vi "welcome.vi"() -> ()   [LabVIEW 2017]
uses:
  GLOBAL/auto.vi
  GLOBAL/all vi close.vi
panel:
  out "first time direct auto":bool
  in  "error in":errorcluster
  in  "EXIT":bool
  in  "PRINTER":bool
  in  "REPORT":bool
  in  "MAIN":bool
  in  "DATA":bool
  in  "USER":bool
  in  "COUNTER":bool
  in  "SETTING":bool
  in  "SHIFT SETTING":bool
  in  "LOGIN":bool
  # "TRACEABILITY"
  # "Powered By- NI Vision, Pune"
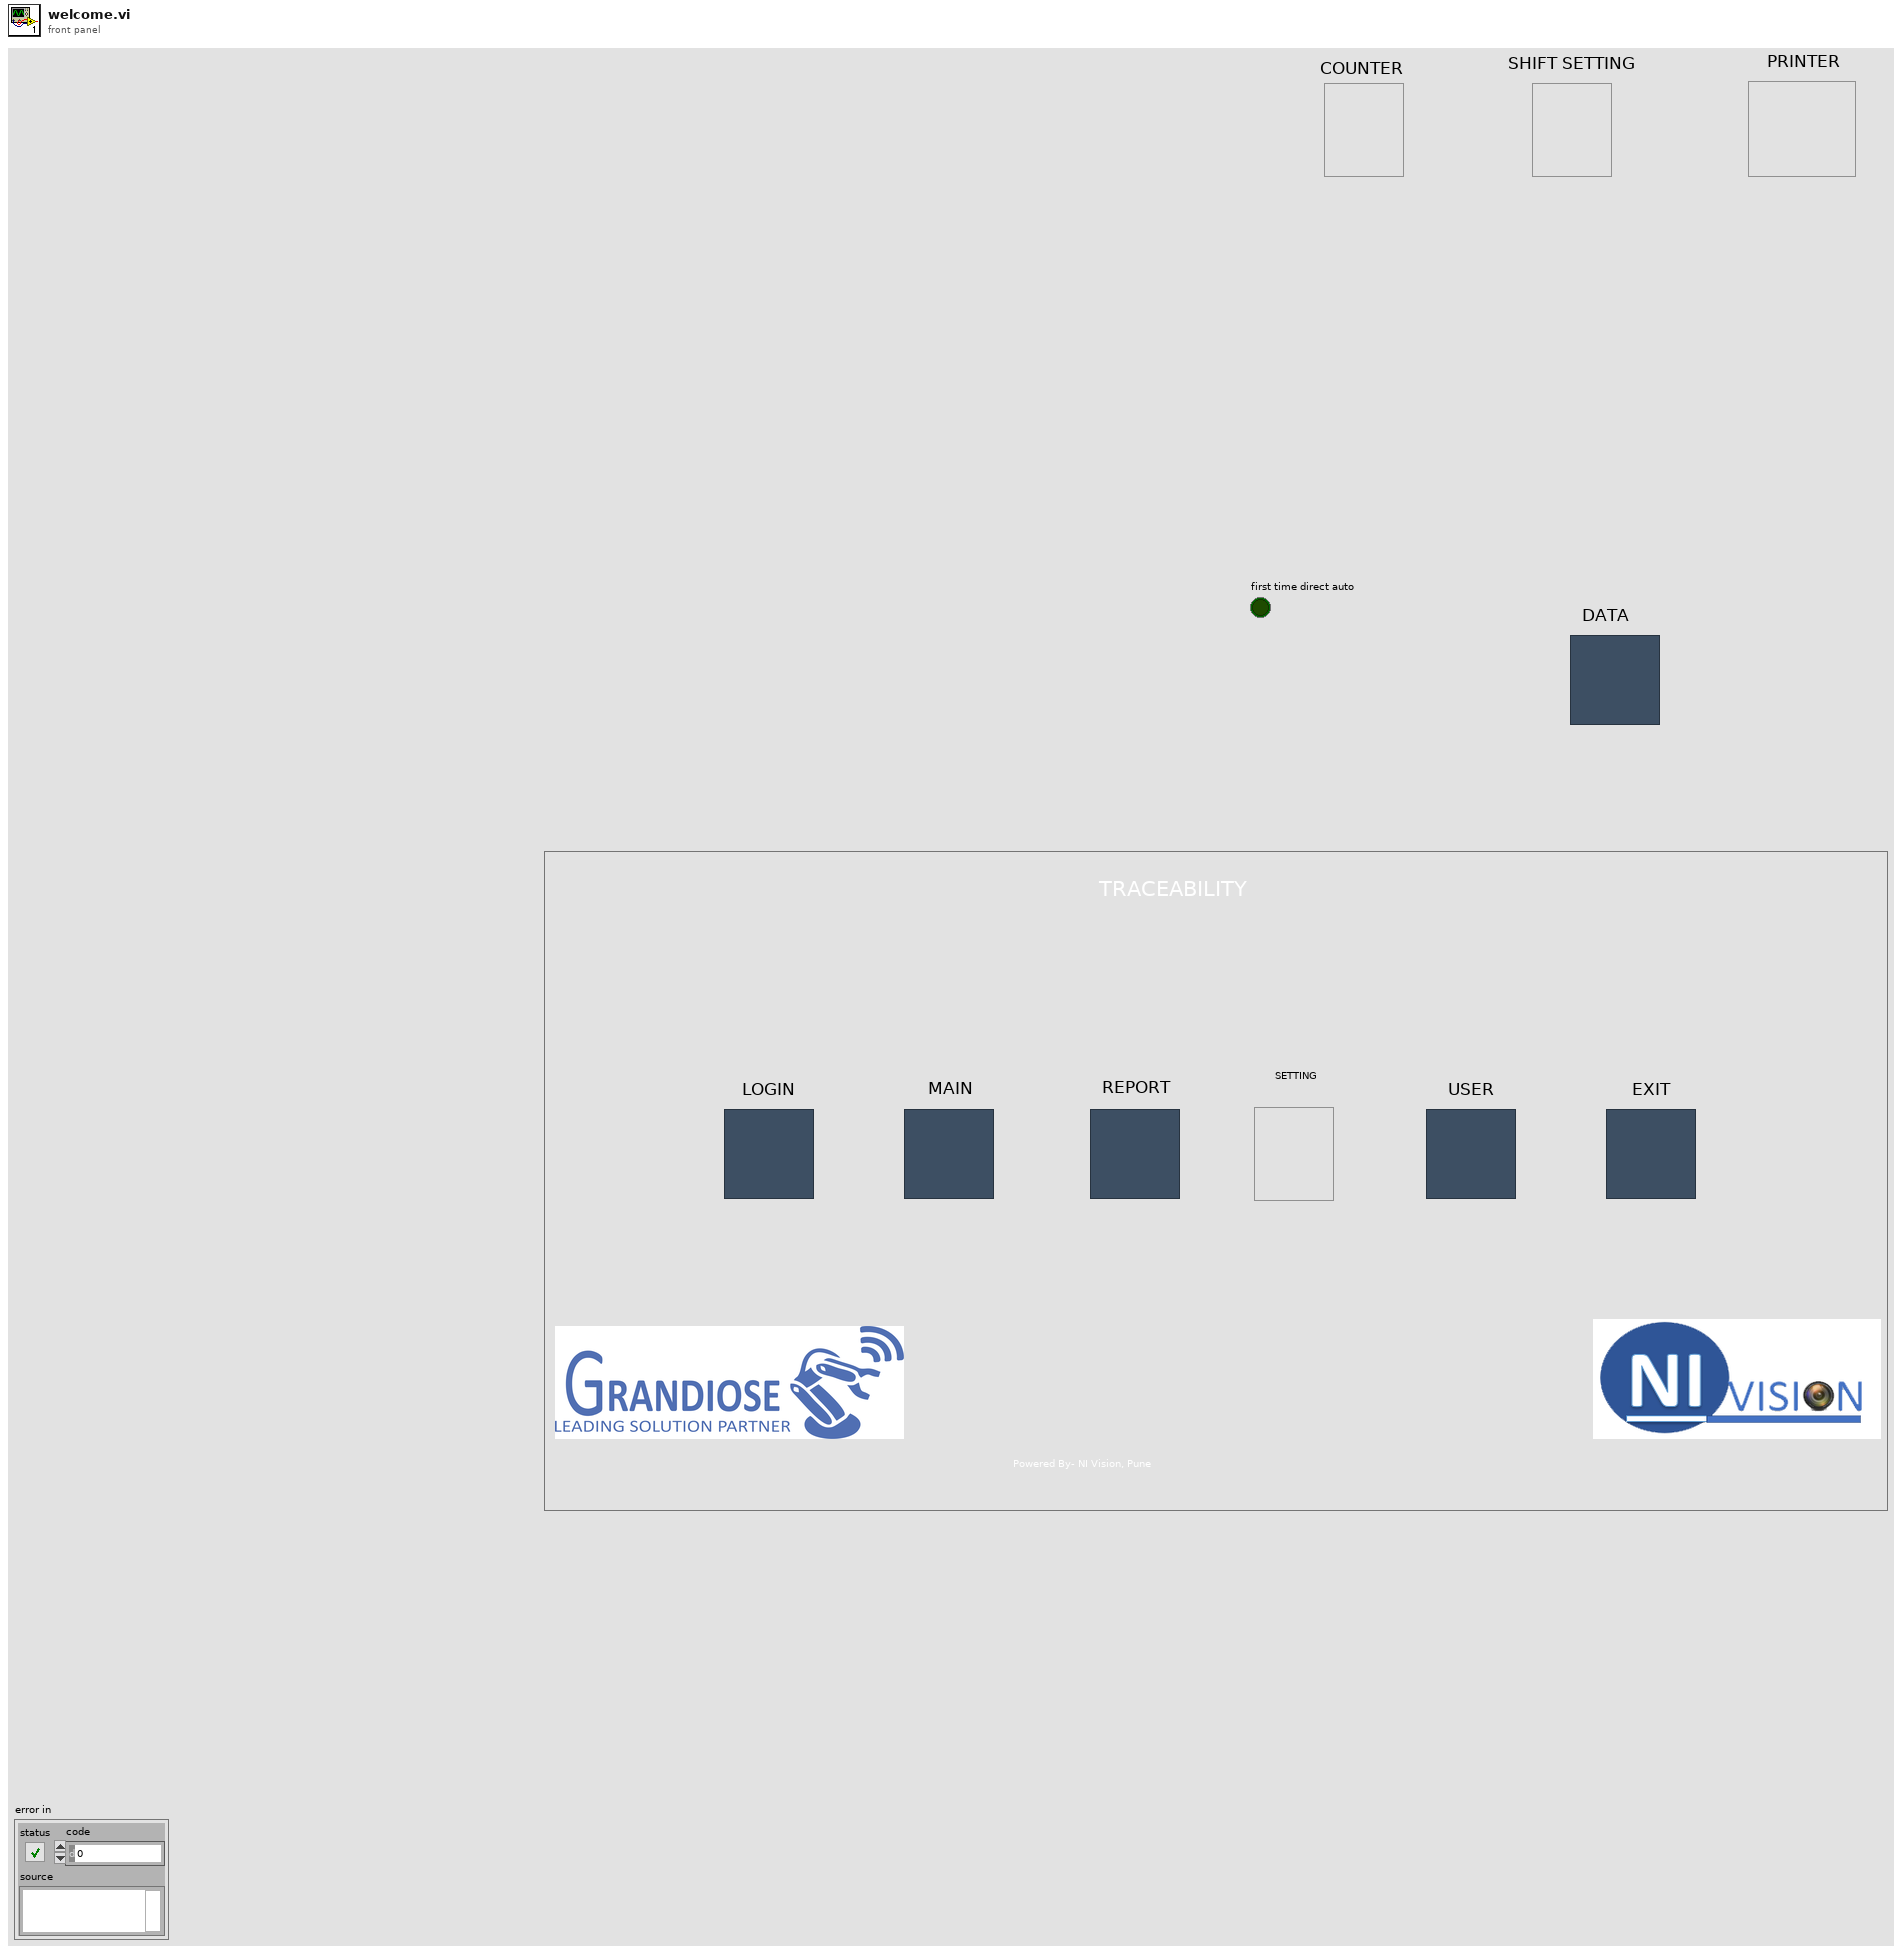
[diagram p1: front panel]
types:
  T1 = enum8{"Enabled", "Disabled", "Disabled and Grayed Out"}
  T2 = enum32{"Invalid", "Standard", "Closed", "Hidden", "Minimized", "Maximized"}
  T3 = enum32{"invalid app kind", "Development System", "Run Time System", "Student Edition", "Embedded LabVIEW", "Evaluation", "Custom"}
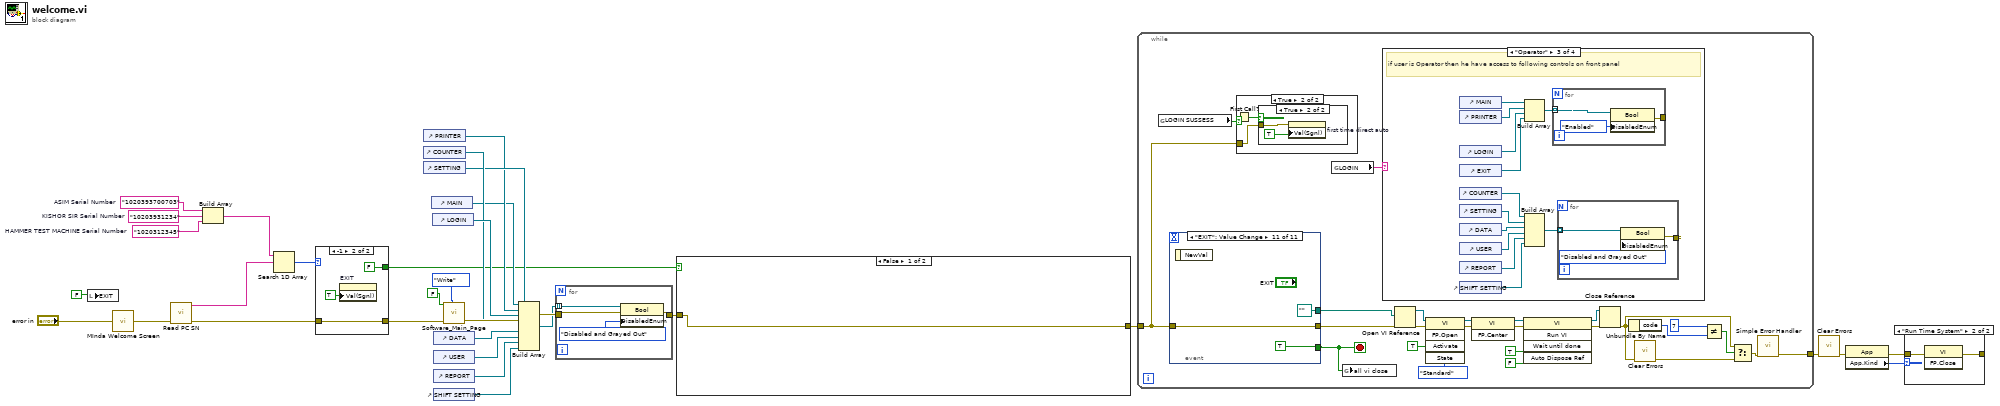
[diagram p0: block diagram]
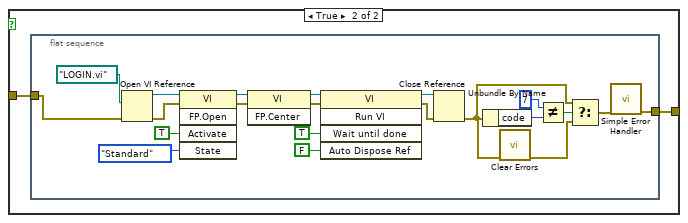
[diagram p2: hidden frame]
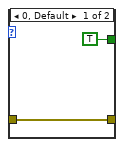
[diagram p3: hidden frame]
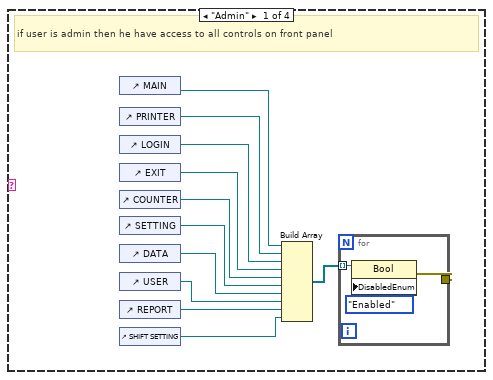
[diagram p7: hidden frame]
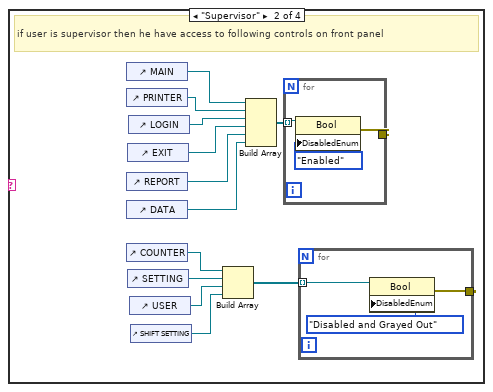
[diagram p8: hidden frame]
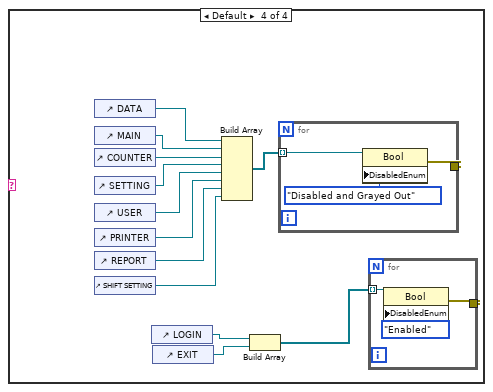
[diagram p9: hidden frame]
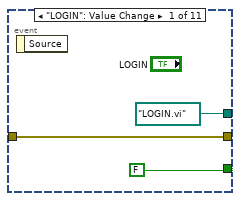
[diagram p10: hidden frame]
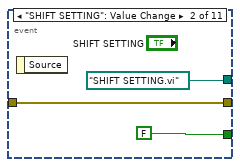
[diagram p11: hidden frame]
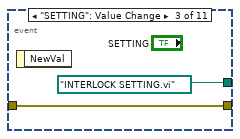
[diagram p12: hidden frame]
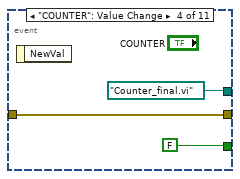
[diagram p13: hidden frame]
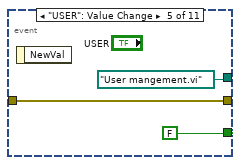
[diagram p14: hidden frame]
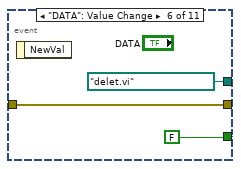
[diagram p15: hidden frame]
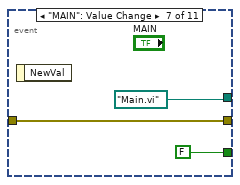
[diagram p16: hidden frame]
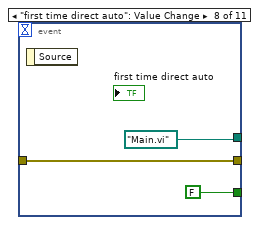
[diagram p17: hidden frame]
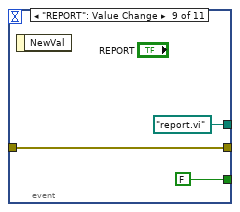
[diagram p18: hidden frame]
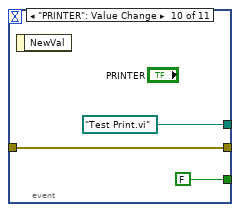
[diagram p19: hidden frame]
diagram:
  w6 = "1020312345"  # HAMMER TEST MACHINE Serial Number
  w7 = "10203931234"  # KISHOR SIR Serial Number
  w8 = "1020393700703"  # ASIM Serial Number
  n1 = local write "EXIT"(FALSE) -> ()
  n2 = call "MInda Welcome Screen.vi"("error in"="error in") -> ("error out"=w10:errorcluster)
  n3 = call "Read PC SN.vi"("error in (no error)"=w10) -> ("error out"=w3:errorcluster, "Serial Number"=w9:string)  [unwired: 9 in]
  n4 = Build Array(w8, w7, w6) -> (w5:string[])
  n5 = Search 1D Array(1D array=w5, element=w9) -> (index of element=w4:i32)  [unwired: 1 in]
  n6 = case shown="-1" w4 {
    tunnel: [w33 w35] -> w2
    tunnel: w3 -> [w33 w35]
    tunnel: [TRUE FALSE] -> w1
    frame 0, Default {
    }
    frame -1 {
      n7 = property on="EXIT" class="Bool (strict)"("Val(Sgnl)"=TRUE) -> ()  [unwired: 2 in, 2 out]
    }
  }
  n8 = control-ref of="PRINTER"() -> (w14:refnum<vi>)
  n9 = control-ref of="COUNTER"() -> (w20:refnum<vi>)
  n10 = control-ref of="SETTING"() -> (w19:refnum<vi>)
  n11 = control-ref of="MAIN"() -> (w13:refnum<vi>)
  n12 = control-ref of="LOGIN"() -> (w21:refnum<vi>)
  n13 = control-ref of="DATA"() -> (w18:refnum<vi>)
  n14 = control-ref of="USER"() -> (w17:refnum<vi>)
  n15 = control-ref of="REPORT"() -> (w16:refnum<vi>)
  n16 = control-ref of="SHIFT SETTING"() -> (w15:refnum<vi>)
  n17 = call "Software_Main_Page.vi"("Enum"=enum16{"Read", "Write"}."Write", "error in (no error)"=w2, "Main_Page_in"=FALSE) -> ("error out"=w23:errorcluster)  [unwired: 7 in, 1 out]
  n18 = Build Array(w13, w14, w21, w20, w19, w18, w17, w16, w15) -> (w22:refnum<vi>[])
  n19 = for {
    tunnel: w22 -> [w40] mode=indexing
    tunnel: w23 -> [w38]
    tunnel: [w37] -> w12
    n20 = property class="Bool"(reference=w40, error in=w38, "DisabledEnum"=T1."Disabled and Grayed Out" ("Disabled")) -> (error out=w37:errorcluster)  [unwired: 1 out]
  }
  n21 = case shown="False" w1 {
    tunnel: [w41 w43] -> w30
    tunnel: w12 -> [w41 w42]
    frame False {
    }
    frame True {
      n22 = flat-sequence {
        tunnel: [w45] -> w43
        tunnel: w42 -> [w44]
        frame #0 {
          n23 = Open VI Reference(vi path=path "LOGIN.vi", error in (no error)=w44) -> (vi reference=w52:refnum<vi>, error out=w64:errorcluster)  [unwired: 4 in]
          n24 = invoke class="VI" method="FP.Open"(reference=w52, error in=w64, "Activate"=TRUE ("Activate?"), "State"=T2."Standard") -> (reference out=w63:refnum<vi>, error out=w58:errorcluster)  [unwired: 1 in, 3 out]
          n25 = invoke class="VI" method="FP.Center"(reference=w63, error in=w58) -> (reference out=w59:refnum<vi>, error out=w60:errorcluster)  [unwired: 1 in, 1 out]
          n26 = invoke class="VI" method="Run VI"(reference=w59, error in=w60, "Wait until done"=TRUE ("Wait Until Done"), "Auto Dispose Ref"=FALSE ("Auto Dispose Reference")) -> (reference out=w61:refnum<vi>, error out=w62:errorcluster)  [unwired: 1 in, 3 out]
          n27 = Close Reference(reference=w61, error in (no error)=w62) -> (error out=w53:errorcluster)
          n28 = Unbundle By Name(w53) -> ("code"=w57:i32)
          n29 = call <vilib>:"Clear Errors.vi"("error in (no error)"=w53) -> ("error out"=w55:errorcluster)  [unwired: 5 in, 1 out]
          n30 = Not Equal?(x=7, y=w57) -> (x != y?=w56:bool)
          n31 = Select(t=w53, s=w56, f=w55) -> (s? t:f=w54:errorcluster)
          n32 = call <vilib>:"Simple Error Handler.vi"("error in (no error)"=w54) -> ("error out"=w45:errorcluster)  [unwired: 4 in, 4 out]
        }
      }
    }
  }
  n33 = while {
    tunnel: w30 -> [w65]
    tunnel: [w69] -> w31
    stop <- w67 stop-if-true
    n34 = global read "auto.vi" "LOGIN SUSSESS"() -> (w66:bool)
    n35 = event shown="[10] \"EXIT\": Value Change" {
      selector: _ -> [_ _ _ _ _ _ _ _ _ _ _]
      dyn-events: _ -> [_ _ _ _ _ _ _ _ _ _ _]
      timeout: _ -> [_ _ _ _ _ _ _ _ _ _ _]
      tunnel: [FALSE FALSE _ FALSE FALSE FALSE FALSE FALSE FALSE FALSE TRUE] -> w67
      tunnel: [path "LOGIN.vi" ("vi path") path "SHIFT SETTING.vi" ("vi path") path "INTERLOCK SETTING.vi" ("vi path") path "Counter_final.vi" ("vi path") path "User mangement.vi" ("vi path") path "delet.vi" ("vi path") path "Main.vi" ("vi path") path "Main.vi" ("vi path") path "report.vi" ("vi path") path "Test Print.vi" ("vi path") path "" ("vi path")] -> w70
      tunnel: w65 -> [w163 w167 w169 w170 w173 w176 w180 w183 w185 w188 w192]
      tunnel: [w163 w167 w169 w170 w173 w176 w180 w183 w185 w188 w192] -> w71
      event "LOGIN": Value Change {
        n36 = event-data() -> ()  [unwired: 1 in, 1 out]
      }
      event "SHIFT SETTING": Value Change {
        n37 = event-data() -> ()  [unwired: 1 in, 1 out]
      }
      event "SETTING": Value Change {
        n38 = event-data() -> ()  [unwired: 1 in, 1 out]
      }
      event "COUNTER": Value Change {
        n39 = event-data() -> ()  [unwired: 1 in, 1 out]
      }
      event "USER": Value Change {
        n40 = event-data() -> ()  [unwired: 1 in, 1 out]
      }
      event "DATA": Value Change {
        n41 = event-data() -> ()  [unwired: 1 in, 1 out]
      }
      event "MAIN": Value Change {
        n42 = event-data() -> ()  [unwired: 1 in, 1 out]
      }
      event "first time direct auto": Value Change {
        n43 = event-data() -> ()  [unwired: 1 in, 1 out]
      }
      event "REPORT": Value Change {
        n44 = event-data() -> ()  [unwired: 1 in, 1 out]
      }
      event "PRINTER": Value Change {
        n45 = event-data() -> ()  [unwired: 1 in, 1 out]
      }
      event "EXIT": Value Change {
        n46 = event-data() -> ()  [unwired: 1 in, 1 out]
      }
    }
    n47 = case shown="True" w66 {
      tunnel: w65 -> [_ w90]
      frame False {
      }
      frame True {
        n48 = First Call?() -> (First Call?: T/F=w91:bool)
        n49 = case shown="True" w91 {
          tunnel: w90 -> [_ w92]
          frame False {
          }
          frame True {
            n50 = property on="first time direct auto" class="Bool (strict)"(error in=w92, "Val(Sgnl)"=TRUE) -> ()  [unwired: 1 in, 2 out]
          }
        }
      }
    }
    n51 = global read "auto.vi" "LOGIN"() -> (w68:string)
    n52 = global write "all vi close.vi" "all vi close"(w67) -> ()
    n53 = case shown="\"Operator\"" w68 {
      frame "Admin" {
        # "if user is admin then he have access to all controls on front panel"
        n54 = control-ref of="MAIN"() -> (w94:refnum<vi>)
        n55 = control-ref of="PRINTER"() -> (w95:refnum<vi>)
        n56 = control-ref of="LOGIN"() -> (w103:refnum<vi>)
        n57 = control-ref of="EXIT"() -> (w102:refnum<vi>)
        n58 = control-ref of="COUNTER"() -> (w101:refnum<vi>)
        n59 = control-ref of="SETTING"() -> (w100:refnum<vi>)
        n60 = control-ref of="DATA"() -> (w99:refnum<vi>)
        n61 = control-ref of="USER"() -> (w98:refnum<vi>)
        n62 = control-ref of="REPORT"() -> (w97:refnum<vi>)
        n63 = control-ref of="SHIFT SETTING"() -> (w96:refnum<vi>)
        n64 = Build Array(w94, w95, w103, w102, w101, w100, w99, w98, w97, w96) -> (w104:refnum<vi>[])
        n65 = for {
          tunnel: w104 -> [w105] mode=indexing
          tunnel: [w106] -> _
          n66 = property class="Bool"(reference=w105, "DisabledEnum"=T1."Enabled" ("Disabled")) -> (error out=w106:errorcluster)  [unwired: 1 in, 1 out]
        }
      }
      frame "Supervisor" {
        # "if user is supervisor then he have access to following controls on front panel"
        n67 = control-ref of="MAIN"() -> (w108:refnum<vi>)
        n68 = control-ref of="PRINTER"() -> (w109:refnum<vi>)
        n69 = control-ref of="REPORT"() -> (w115:refnum<vi>)
        n70 = control-ref of="DATA"() -> (w114:refnum<vi>)
        n71 = control-ref of="COUNTER"() -> (w113:refnum<vi>)
        n72 = control-ref of="EXIT"() -> (w116:refnum<vi>)
        n73 = control-ref of="SETTING"() -> (w112:refnum<vi>)
        n74 = control-ref of="LOGIN"() -> (w117:refnum<vi>)
        n75 = control-ref of="USER"() -> (w111:refnum<vi>)
        n76 = control-ref of="SHIFT SETTING"() -> (w110:refnum<vi>)
        n77 = Build Array(w113, w112, w111, w110) -> (w118:refnum<vi>[])
        n78 = Build Array(w108, w109, w117, w116, w115, w114) -> (w119:refnum<vi>[])
        n79 = for {
          tunnel: w119 -> [w123] mode=indexing
          tunnel: [w124] -> _
          n80 = property class="Bool"(reference=w123, "DisabledEnum"=T1."Enabled" ("Disabled")) -> (error out=w124:errorcluster)  [unwired: 1 in, 1 out]
        }
        n81 = for {
          tunnel: [w121] -> _
          tunnel: w118 -> [w120] mode=indexing
          n82 = property class="Bool"(reference=w120, "DisabledEnum"=T1."Disabled and Grayed Out" ("Disabled")) -> (error out=w121:errorcluster)  [unwired: 1 in, 1 out]
        }
      }
      frame "Operator" {
        # "if user is Operator then he have access to following controls on front panel"
        n83 = control-ref of="MAIN"() -> (w126:refnum<vi>)
        n84 = control-ref of="PRINTER"() -> (w135:refnum<vi>)
        n85 = control-ref of="LOGIN"() -> (w128:refnum<vi>)
        n86 = control-ref of="EXIT"() -> (w127:refnum<vi>)
        n87 = control-ref of="COUNTER"() -> (w129:refnum<vi>)
        n88 = control-ref of="SETTING"() -> (w134:refnum<vi>)
        n89 = control-ref of="DATA"() -> (w133:refnum<vi>)
        n90 = control-ref of="USER"() -> (w132:refnum<vi>)
        n91 = control-ref of="REPORT"() -> (w131:refnum<vi>)
        n92 = control-ref of="SHIFT SETTING"() -> (w130:refnum<vi>)
        n93 = Build Array(w126, w135, w128, w127) -> (w137:refnum<vi>[])
        n94 = Build Array(w129, w134, w133, w132, w131, w130) -> (w136:refnum<vi>[])
        n95 = for {
          tunnel: w137 -> [w143] mode=indexing
          tunnel: [w141] -> _
          n96 = property class="Bool"(reference=w143, "DisabledEnum"=T1."Enabled" ("Disabled")) -> (error out=w141:errorcluster)  [unwired: 1 in, 1 out]
        }
        n97 = for {
          tunnel: w136 -> [w140] mode=indexing
          tunnel: [w138] -> _
          n98 = property class="Bool"(reference=w140, "DisabledEnum"=T1."Disabled and Grayed Out" ("Disabled")) -> (error out=w138:errorcluster)  [unwired: 1 in, 1 out]
        }
      }
      frame Default {
        n99 = control-ref of="DATA"() -> (w148:refnum<vi>)
        n100 = control-ref of="MAIN"() -> (w147:refnum<vi>)
        n101 = control-ref of="COUNTER"() -> (w149:refnum<vi>)
        n102 = control-ref of="SETTING"() -> (w150:refnum<vi>)
        n103 = control-ref of="USER"() -> (w151:refnum<vi>)
        n104 = control-ref of="PRINTER"() -> (w152:refnum<vi>)
        n105 = control-ref of="REPORT"() -> (w153:refnum<vi>)
        n106 = control-ref of="SHIFT SETTING"() -> (w154:refnum<vi>)
        n107 = control-ref of="LOGIN"() -> (w144:refnum<vi>)
        n108 = control-ref of="EXIT"() -> (w146:refnum<vi>)
        n109 = Build Array(w148, w147, w149, w150, w151, w152, w153, w154) -> (w155:refnum<vi>[])
        n110 = Build Array(w144, w146) -> (w145:refnum<vi>[])
        n111 = for {
          tunnel: w155 -> [w159] mode=indexing
          tunnel: [w160] -> _
          n112 = property class="Bool"(reference=w159, "DisabledEnum"=T1."Disabled and Grayed Out" ("Disabled")) -> (error out=w160:errorcluster)  [unwired: 1 in, 1 out]
        }
        n113 = for {
          tunnel: w145 -> [w156] mode=indexing
          tunnel: [w157] -> _
          n114 = property class="Bool"(reference=w156, "DisabledEnum"=T1."Enabled" ("Disabled")) -> (error out=w157:errorcluster)  [unwired: 1 in, 1 out]
        }
      }
    }
    n115 = Open VI Reference(vi path=w70, error in (no error)=w71) -> (vi reference=w89:refnum<vi>, error out=w78:errorcluster)  [unwired: 4 in]
    n116 = invoke class="VI" method="FP.Open"(reference=w89, error in=w78, "Activate"=TRUE ("Activate?"), "State"=T2."Standard") -> (reference out=w79:refnum<vi>, error out=w84:errorcluster)  [unwired: 1 in, 3 out]
    n117 = invoke class="VI" method="FP.Center"(reference=w79, error in=w84) -> (reference out=w83:refnum<vi>, error out=w82:errorcluster)  [unwired: 1 in, 1 out]
    n118 = invoke class="VI" method="Run VI"(reference=w83, error in=w82, "Wait until done"=TRUE ("Wait Until Done"), "Auto Dispose Ref"=FALSE ("Auto Dispose Reference")) -> (reference out=w81:refnum<vi>, error out=w80:errorcluster)  [unwired: 1 in, 3 out]
    n119 = Close Reference(reference=w81, error in (no error)=w80) -> (error out=w77:errorcluster)
    n120 = Unbundle By Name(w77) -> ("code"=w85:i32)
    n121 = call <vilib>:"Clear Errors.vi"("error in (no error)"=w77) -> ("error out"=w87:errorcluster)  [unwired: 5 in, 1 out]
    n122 = Not Equal?(x=7, y=w85) -> (x != y?=w86:bool)
    n123 = Select(t=w77, s=w86, f=w87) -> (s? t:f=w88:errorcluster)
    n124 = call <vilib>:"Simple Error Handler.vi"("error in (no error)"=w88) -> ("error out"=w69:errorcluster)  [unwired: 4 in, 4 out]
  }
  n125 = call <vilib>:"Clear Errors.vi"("error in (no error)"=w31) -> ("error out"=w27:errorcluster)  [unwired: 5 in, 1 out]
  n126 = property class="App"(error in=w27) -> (error out=w28:errorcluster, "App.Kind"=w29:T3)  [unwired: 1 in, 1 out]
  n127 = case shown="\"Run Time System\"" w29 {
    tunnel: w28 -> [w194 w196]
    tunnel: [w194 w195] -> _
    frame Default {
    }
    frame "Run Time System" {
      n128 = invoke class="VI" method="FP.Close"(error in=w196) -> (error out=w195:errorcluster)  [unwired: 2 in, 2 out]
    }
  }
